vi "FGV_Configuration.vi"(5 "Configuration File Path":path=path "D:/raw", 7 "Action_Data":T1(ring), 8 "error in":errorcluster, 10 "Data In":cluster{"Data name":string, "Data":variant}, 11 "KeyName":string) -> (0 "error out":errorcluster, 2 "Data Array out":cluster{"Data name":string, "Data":variant}[](array[cluster]), 3 "Data  Out":cluster{"Data name":string, "Data":variant})   [LabVIEW 2015]
uses:
  <vilib>/Utility/config.llb/Read Key (String).vi
  <vilib>/Utility/config.llb/Write Key (String).vi
  <vilib>/Utility/config.llb/NI_LVConfig.lvlib
panel:
  out "Section Array out":string[][](array[string])
  in  "Section":string="Section"
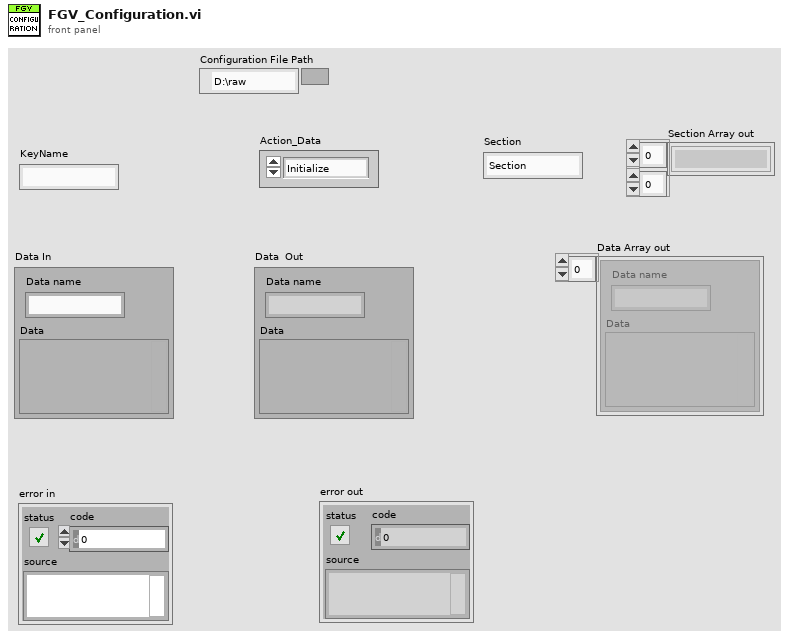
[diagram p1: front panel]
types:
  T1 = enum16{"Initialize", "OpenFile", "Load Data", "Get Data", "Set Data", "Delete Data", "Close", "Idle"}
  T2 = typedef "NI_LVConfig.lvlib/Config Data RefNum.ctl" = refnum<k1>
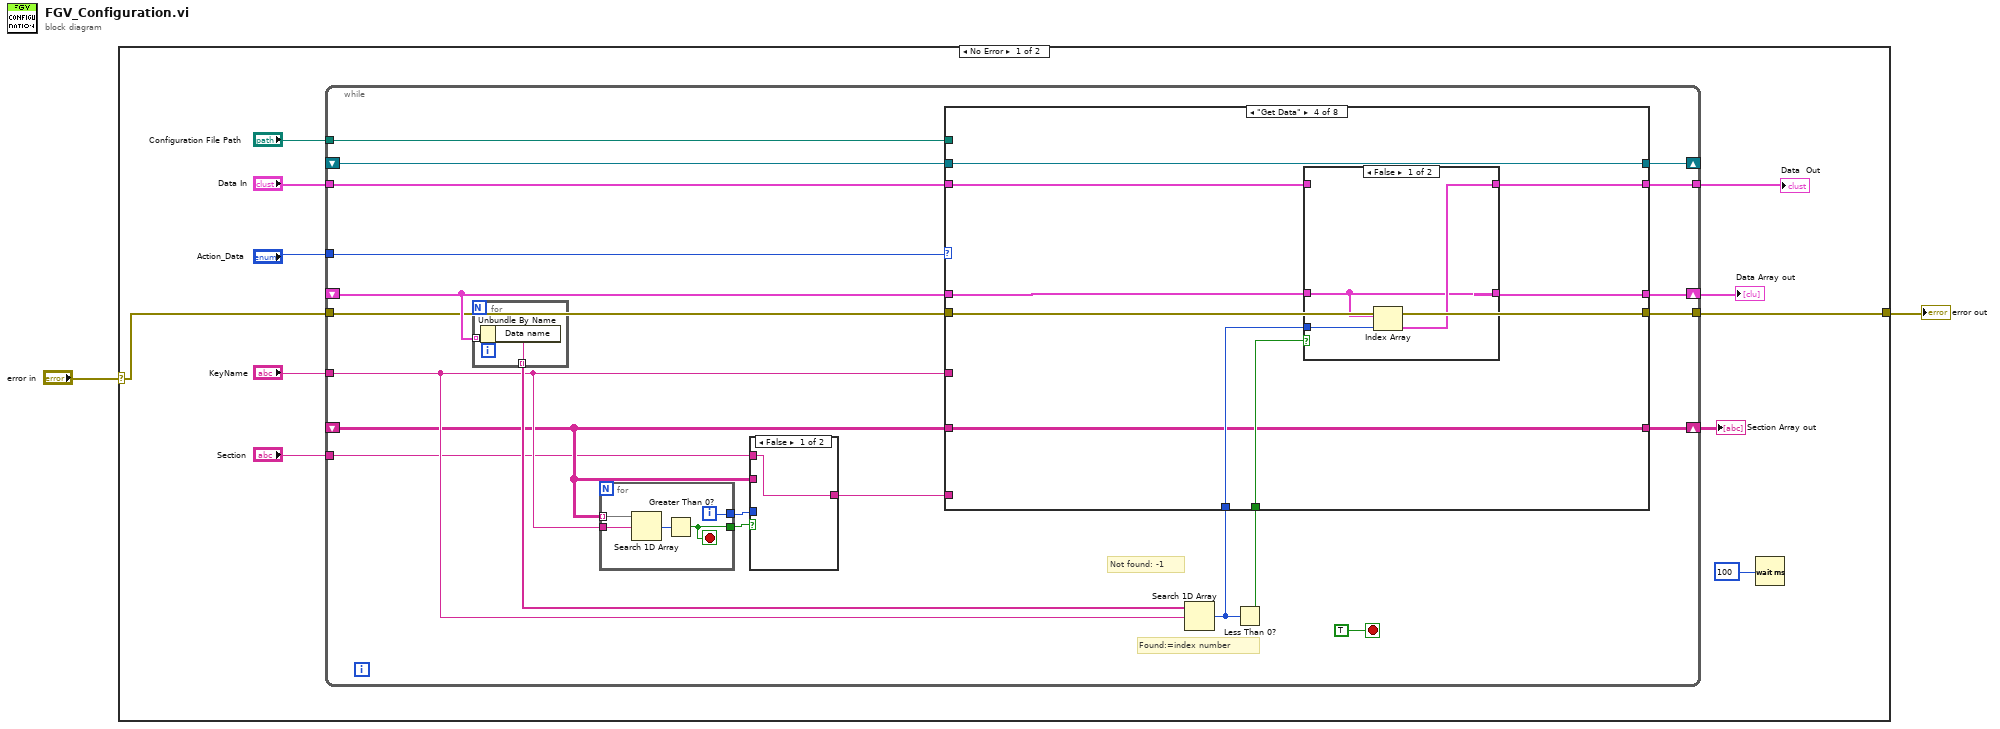
[diagram p0: block diagram]
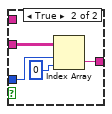
[diagram p2: hidden frame]
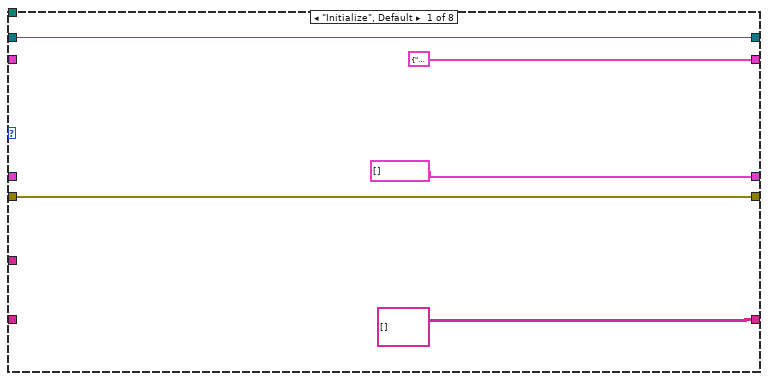
[diagram p3: hidden frame]
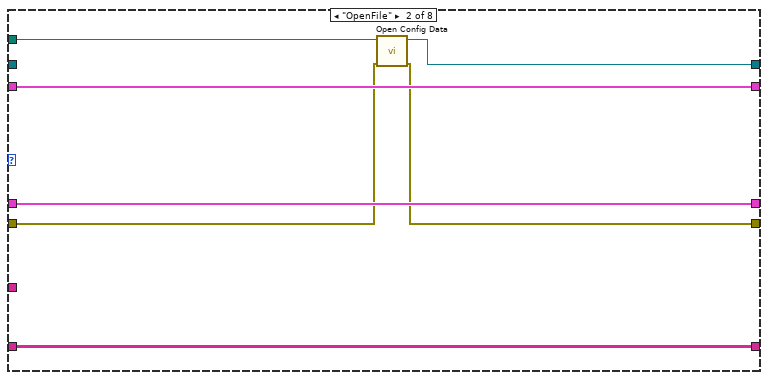
[diagram p4: hidden frame]
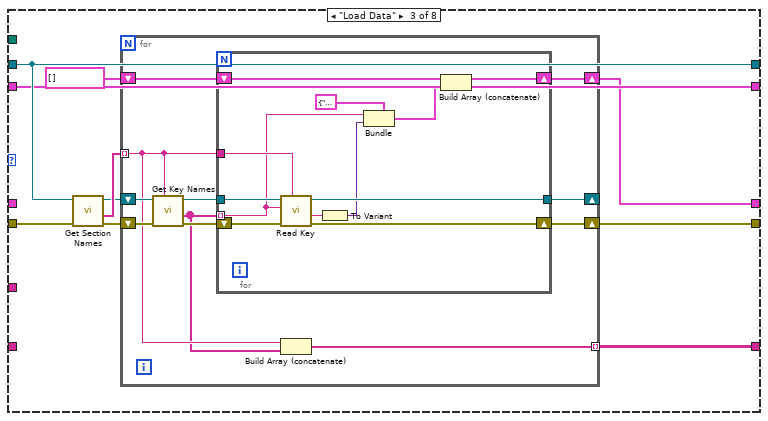
[diagram p5: hidden frame]
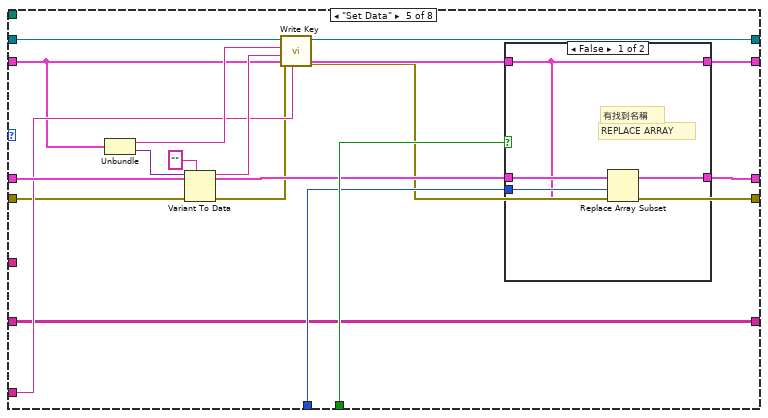
[diagram p7: hidden frame]
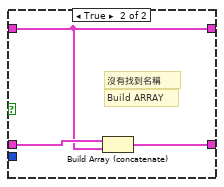
[diagram p8: hidden frame]
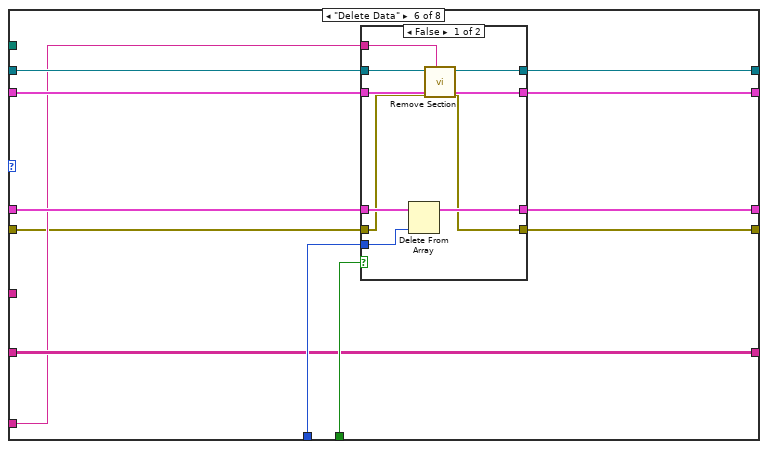
[diagram p9: hidden frame]
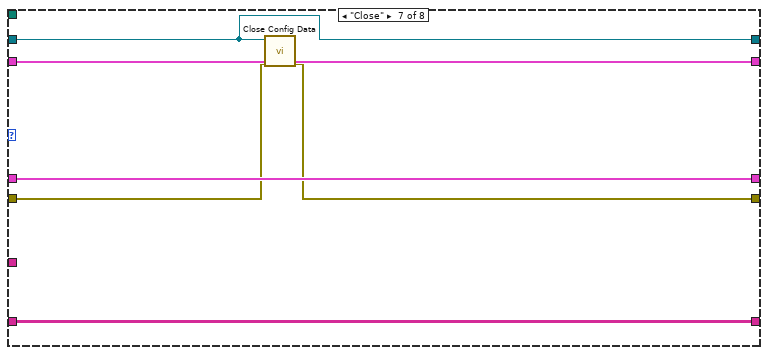
[diagram p11: hidden frame]
diagram:
  n1 = case shown="No Error" "error in" {
    selector: "error in" -> [w4 w166]
    tunnel: [w3 w166] -> w1
    frame No Error {
      n2 = while {
        tunnel: "Action_Data" -> [w34]
        tunnel: "Data In" -> [w32]
        tunnel: [w31] -> w10
        shift-right: [w30] -> w9
        shift-left: _ -> [w29]
        tunnel: "KeyName" -> [w19]
        tunnel: "Configuration File Path" -> [w25]
        shift-right: [w24] -> _
        shift-left: _ -> [w23]
        tunnel: "Section" -> [w16]
        shift-right: [w22] -> w5
        shift-left: _ -> [w18]
        tunnel: w4 -> [w15]
        tunnel: [w14] -> w3
        stop <- TRUE stop-if-true
        # "Not found: -1"
        # "Found:=index number"
        n3 = for {
          tunnel: w29 -> [w46] mode=indexing
          tunnel: [w45] -> w28 mode=indexing
          n4 = Unbundle By Name(w46) -> ("Data name"=w45:string)
        }
        n5 = for {
          tunnel: w18 -> [w44] mode=indexing
          tunnel: w19 -> [w43]
          tunnel: [w41] -> w21
          tunnel: [w40] -> w20
          i -> [w41]
          stop <- w40 stop-if-true
          n6 = Search 1D Array(1D array=w44, element=w43) -> (index of element=w42:i32)  [unwired: 1 in]
          n7 = Greater Than 0?(x=w42) -> (x > 0?=w40:bool)
        }
        n8 = case shown="False" w20 {
          tunnel: w18 -> [_ w39]
          tunnel: w21 -> [_ w38]
          tunnel: [w35 w36] -> w17
          tunnel: w16 -> [w35 _]
          frame False {
          }
          frame True {
            n9 = Index Array(array=w39, index (row)=w38, index (col)=0 ("disabled index (col)")) -> (element=w36:string)
          }
        }
        n10 = Search 1D Array(1D array=w28, element=w19) -> (index of element=w26:i32)  [unwired: 1 in]
        n11 = Less Than 0?(x=w26) -> (x < 0?=w27:bool)
        n12 = case shown="\"Get Data\"" w34 {
          tunnel: w32 -> [_ w55 w63 w95 w109 w136 w160 w165]
          tunnel: [cluster{"Data name":string, "Data":variant} {"Data name"="", "Data"=variant} ("Data In") w55 w63 w97 w117 w137 w160 w165] -> w31
          tunnel: [cluster{"Data name":string, "Data":variant}[] [] w54 w62 w96 w119 w138 w159 w164] -> w30
          tunnel: w29 -> [_ w54 _ w99 w120 w140 w159 w164]
          tunnel: w27 -> [_ _ _ w100 w122 w141 _ _]
          tunnel: w26 -> [_ _ _ w98 w121 w139 _ _]
          tunnel: w25 -> [_ w56 _ _ _ _ _ _]
          tunnel: [w48 w57 w64 w94 w112 w134 w157 w163] -> w24
          tunnel: w23 -> [w48 _ w64 w94 w118 w135 w157 w163]
          tunnel: [string[][] [] w58 w61 w93 w110 w133 w158 w162] -> w22
          tunnel: w18 -> [_ w58 _ w93 w110 w133 w158 w162]
          tunnel: w19 -> [_ _ _ _ _ _ _ _]
          tunnel: w17 -> [_ _ _ _ w111 w132 _ _]
          tunnel: w15 -> [w47 w53 w60 w92 w108 w131 w156 w161]
          tunnel: [w47 w52 w59 w92 w106 w130 w155 w161] -> w14
          frame "Initialize", Default {
          }
          frame "OpenFile" {
            n13 = call <vilib>:"Open Config Data.vi"("error in (no error)"=w53, "configuration file path"=w56) -> ("error out"=w52:errorcluster, "refnum"=w57:T2)  [unwired: 7 in, 1 out]
          }
          frame "Load Data" {
            n14 = call <vilib>:"Get Section Names.vi"("error in (no error)"=w60, "refnum"=w64) -> ("error out"=w66:errorcluster, "section names"=w67:string[], "refnum out"=w65:T2)  [unwired: 7 in]
            n15 = for {
              shift-right: [w77] -> _
              shift-left: w65 -> [w75]
              shift-right: [w79] -> w59
              shift-left: w66 -> [w74]
              tunnel: w67 -> [w71] mode=indexing
              shift-right: [w73] -> w62
              shift-left: cluster{"Data name":string, "Data":variant}[] [] -> [w72]
              tunnel: [w69] -> w61 mode=indexing
              n16 = call <vilib>:"Get Key Names.vi"("section"=w71, "error in (no error)"=w74, "refnum"=w75) -> ("error out"=w78:errorcluster, "key names"=w70:string[], "refnum out"=w76:T2)  [unwired: 5 in, 1 out]
              n17 = for {
                tunnel: w76 -> [w91]
                tunnel: w71 -> [w90]
                shift-right: [w89] -> w79
                shift-left: w78 -> [w88]
                tunnel: w70 -> [w85] mode=indexing
                tunnel: [w87] -> w77
                shift-right: [w80] -> w73
                shift-left: w72 -> [w81]
                n18 = call-poly <vilib>:"Read Key.vi"("section"=w90, "error in (no error)"=w88, "key"=w85, "refnum"=w91) -> ("error out"=w89:errorcluster, "value"=w86:string, "refnum out"=w87:T2)  [unwired: 4 in, 1 out]
                n19 = To Variant(anything=w86) -> (Variant=w84:variant)
                n20 = Bundle(cluster=cluster{"Data name":string, "Data":variant} {"Data name"="", "Data"=variant} ("Data  Out"), "Data name"=w85, "Data"=w84) -> (w82:cluster{"Data name":string, "Data":variant})
                n21 = Build Array (concatenate)(w81, w82) -> (w80:cluster{"Data name":string, "Data":variant}[])
              }
              n22 = Build Array (concatenate)(w71, w70) -> (w69:string[])
            }
          }
          frame "Get Data" {
            n23 = case shown="False" w100 {
              tunnel: w99 -> [w101 w105]
              tunnel: w98 -> [w103 _]
              tunnel: [w102 w104] -> w97
              tunnel: [w101 w105] -> w96
              tunnel: w95 -> [_ w104]
              frame False {
                n24 = Index Array(array=w101, index=w103) -> (element=w102:cluster{"Data name":string, "Data":variant})
              }
              frame True {
              }
            }
          }
          frame "Set Data" {
            n25 = Unbundle(w109) -> ("Data name"=w113:string, "Data"=w116:variant)
            n26 = Variant To Data(error in=w108, type="", Variant=w116) -> (data=w114:string, error out=w107:errorcluster)
            n27 = call-poly <vilib>:"Write Key.vi"("section"=w111, "error in (no error)"=w107, "value"=w114, "key"=w113, "refnum"=w118) -> ("error out"=w106:errorcluster, "refnum out"=w112:T2)  [unwired: 4 in, 1 out]
            n28 = case shown="False" w122 {
              tunnel: w121 -> [w126 _]
              tunnel: w120 -> [w124 w129]
              tunnel: [w125 w128] -> w119
              tunnel: [w123 w127] -> w117
              tunnel: w109 -> [w123 w127]
              frame False {
                # "REPLACE ARRAY"
                # "有找到名稱"
                n29 = Replace Array Subset(array=w124, new element=w123, index=w126) -> (w125:cluster{"Data name":string, "Data":variant}[])
              }
              frame True {
                # "Build ARRAY"
                # "沒有找到名稱"
                n30 = Build Array (concatenate)(w129, w127) -> (w128:cluster{"Data name":string, "Data":variant}[])
              }
            }
          }
          frame "Delete Data" {
            n31 = case shown="False" w141 {
              tunnel: w140 -> [w150 w154]
              tunnel: w139 -> [w147 _]
              tunnel: [w149 w154] -> w138
              tunnel: [w148 w153] -> w137
              tunnel: w136 -> [w148 w153]
              tunnel: w135 -> [w146 w152]
              tunnel: [w145 w152] -> w134
              tunnel: w132 -> [w144 _]
              tunnel: w131 -> [w143 w151]
              tunnel: [w142 w151] -> w130
              frame False {
                n32 = Delete From Array(array=w150, index=w147) -> (array with subset deleted=w149:cluster{"Data name":string, "Data":variant}[])  [unwired: 1 in, 1 out]
                n33 = call <vilib>:"Remove Section.vi"("section"=w144, "error in (no error)"=w143, "refnum"=w146) -> ("error out"=w142:errorcluster, "refnum out"=w145:T2)  [unwired: 6 in, 1 out]
              }
              frame True {
              }
            }
          }
          frame "Close" {
            n34 = call <vilib>:"Close Config Data.vi"("error in (no error)"=w156, "refnum"=w157) -> ("error out"=w155:errorcluster)  [unwired: 8 in, 1 out]
          }
          frame "Idle" {
          }
        }
      }
      "Data  Out" <- w10
      "Data Array out" <- w9
      "Section Array out" <- w5
      n35 = Wait (ms)(milliseconds to wait=u32 100) -> ()  [unwired: 1 out]
    }
    frame Error {
    }
  }
  "error out" <- w1
